vi "Create.vi"(10 "Status Notifier":refnum<notifier>) -> (3 "System Config Status API out":refnum<class "System Config Status API.lvclass">)   [LabVIEW 2020, in "Volatus.lvlib" / "System Config Status API.lvclass"]
uses:
  System Config Status API.lvclass
  System Config Status API.lvclass/System Config Status API.ctl
  Config Alert Module/Node Config Info.ctl
  Volatus.lvlib
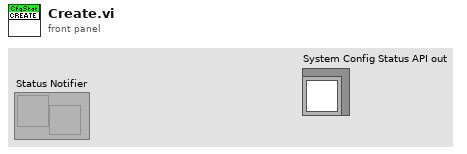
[diagram p1: front panel]
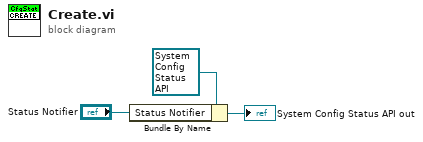
[diagram p0: block diagram]
diagram:
  n1 = Bundle By Name(cluster=refnum<class "System Config Status API.lvclass"> refnum ("System Config Status API in"), "Status Notifier"="Status Notifier") -> (→"System Config Status API out":refnum<class "System Config Status API.lvclass">)
